vi "Determine Waveform Header.vi"(8 "error in (no error)":errorcluster, 10 "Waveform Settings":T1, 11 "Model in":refnum<class "Model.lvclass">) -> (0 "error out":errorcluster, 2 "Waveform Header":string, 3 "Model out":refnum<class "Model.lvclass">)   [LabVIEW 2015, in "Model.lvclass"]
uses:
  Model.lvclass
  Typedefs/Waveform Settings.ctl
  Typedefs/Waveform Types.ctl
  Typedefs/FAMT Typedefs.lvlib
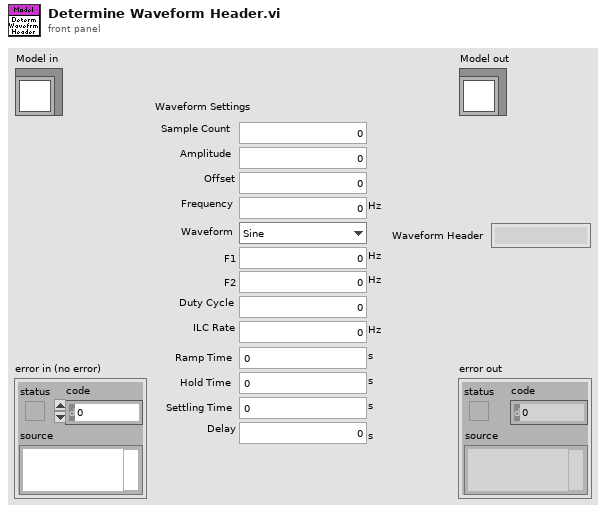
[diagram p1: front panel]
types:
  T1 = typedef "FAMT Typedefs.lvlib/Waveform Settings.ctl" = cluster{"Sample Count":u32, "Amplitude":dbl, "Offset":dbl, "Frequency":dbl[unit], "Waveform":T2, "F1":dbl[unit], "F2":dbl[unit], "Duty Cycle":dbl, "ILC Rate":dbl[unit], "Ramp Time":dbl[unit], "Hold Time":dbl[unit], "Settling Time":dbl[unit], "Delay":dbl[unit]}
  T2 = typedef "FAMT Typedefs.lvlib/Waveform Types.ctl" = enum16{"Sine", "Triangle", "Square", "Sawtooth", "Chirp", "Gaussian", "Trapezoid"}
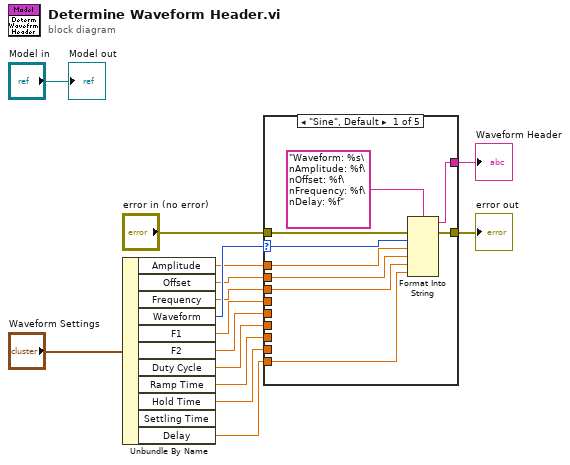
[diagram p0: block diagram]
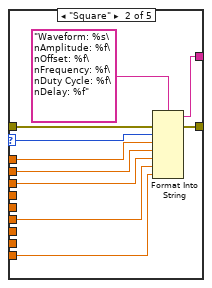
[diagram p2: hidden frame]
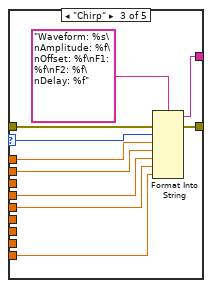
[diagram p3: hidden frame]
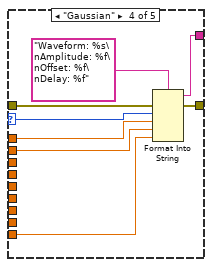
[diagram p4: hidden frame]
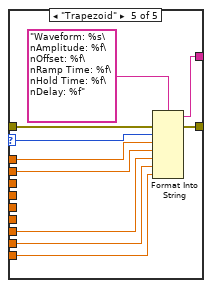
[diagram p5: hidden frame]
diagram:
  n1 = Unbundle By Name("Waveform Settings") -> ("Amplitude"=w10:dbl, "Offset"=w9:dbl, "Frequency"=w8:dbl[unit], "Waveform"=w13:T2, "F1"=w5:dbl[unit], "F2"=w4:dbl[unit], "Duty Cycle"=w6:dbl, "Ramp Time"=w3:dbl[unit], "Hold Time"=w2:dbl[unit], "Delay"=w7:dbl[unit])  [unwired: 1 out]
  n2 = case shown="\"Sine\", Default" w13 {
    selector: w13 -> [w20 w32 w43 w48 w58]
    tunnel: [w23 w25 w35 w52 w61] -> w1
    tunnel: "error in (no error)" -> [w22 w27 w37 w50 w59]
    tunnel: [w21 w26 w36 w51 w60] -> w11
    tunnel: w10 -> [w19 w31 w42 w47 w57]
    tunnel: w9 -> [w18 w30 w41 w46 w56]
    tunnel: w8 -> [w17 w29 _ _ _]
    tunnel: w7 -> [w16 w33 w38 w45 w53]
    tunnel: w6 -> [_ w28 _ _ _]
    tunnel: w5 -> [_ _ w40 _ _]
    tunnel: w4 -> [_ _ w39 _ _]
    tunnel: w3 -> [_ _ _ _ w55]
    tunnel: w2 -> [_ _ _ _ w54]
    frame "Sine", Default {
      n3 = Format Into String(format string="Waveform: %s\nAmplitude: %f\nOffset: %f\nFrequency: %f\nDelay: %f", error in=w22, w20, w19, w18, w17, w16) -> (resulting string=w23:string, error out=w21:errorcluster)  [unwired: 1 in]
    }
    frame "Square" {
      n4 = Format Into String(format string="Waveform: %s\nAmplitude: %f\nOffset: %f\nFrequency: %f\nDuty Cycle: %f\nDelay: %f", error in=w27, w32, w31, w30, w29, w28, w33) -> (resulting string=w25:string, error out=w26:errorcluster)  [unwired: 1 in]
    }
    frame "Chirp" {
      n5 = Format Into String(format string="Waveform: %s\nAmplitude: %f\nOffset: %f\nF1: %f\nF2: %f\nDelay: %f", error in=w37, w43, w42, w41, w40, w39, w38) -> (resulting string=w35:string, error out=w36:errorcluster)  [unwired: 1 in]
    }
    frame "Gaussian" {
      n6 = Format Into String(format string="Waveform: %s\nAmplitude: %f\nOffset: %f\nDelay: %f", error in=w50, w48, w47, w46, w45) -> (resulting string=w52:string, error out=w51:errorcluster)  [unwired: 1 in]
    }
    frame "Trapezoid" {
      n7 = Format Into String(format string="Waveform: %s\nAmplitude: %f\nOffset: %f\nRamp Time: %f\nHold Time: %f\nDelay: %f", error in=w59, w58, w57, w56, w55, w54, w53) -> (resulting string=w61:string, error out=w60:errorcluster)  [unwired: 1 in]
    }
  }
  "error out" <- w11
  "Waveform Header" <- w1
  "Model out" <- "Model in"
